vi "task3.vi"() -> ()   [LabVIEW 2021]
panel:
  out "Phase, Freq":cluster{i32[], "detected phases (deg)":dbl[]}(graph)
  out "Amp, Freq":cluster{i32[], dbl[]}(graph)
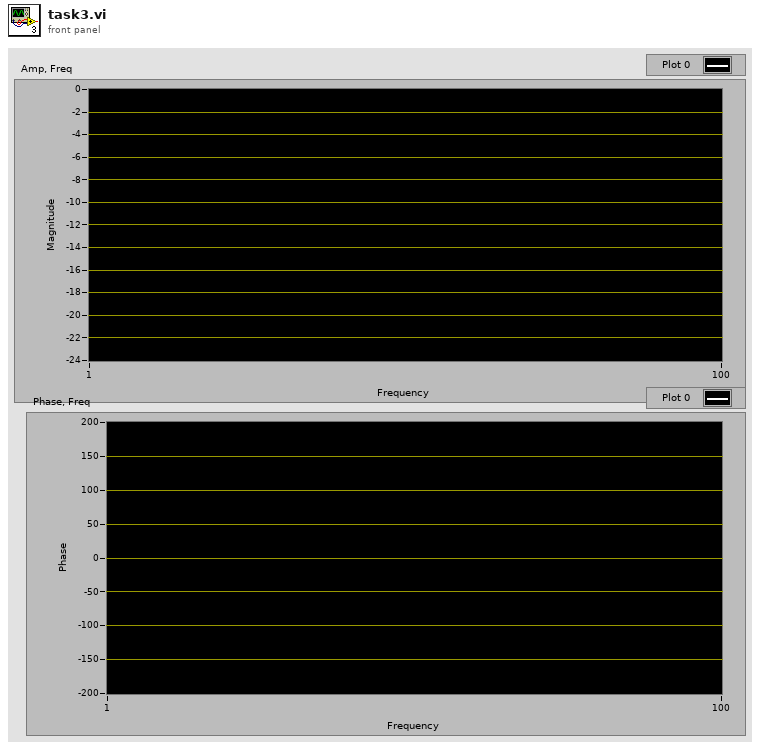
[diagram p1: front panel]
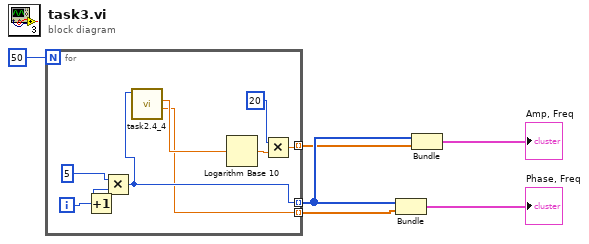
[diagram p0: block diagram]
diagram:
  n1 = for {
    N: 50 -> [_]
    tunnel: [w9] -> w5 mode=indexing
    tunnel: [w10] -> w3 mode=indexing
    tunnel: [w7] -> w2 mode=indexing
    i -> [w15]
    n2 = Increment(x=w15) -> (x+1=w14:i32)
    n3 = Multiply(x=5, y=w14) -> (x*y=w9:i32)
    n4 = call "task2.4_4.vi"("Frequency"=w9) -> ("A1 phase (deg)"=w7:dbl, "A1 amplitude (db)"=w8:dbl)  [unwired: 8 in, 1 out]
    n5 = Logarithm Base 10(1:w8) -> (0:w12:dbl)
    n6 = Multiply(x=20, y=w12) -> (x*y=w10:dbl)
  }
  n7 = Bundle(w5, w2) -> (→"Phase, Freq":cluster{i32[], dbl[]})  [unwired: 1 in]
  n8 = Bundle(w5, w3) -> (→"Amp, Freq":cluster{i32[], dbl[]})  [unwired: 1 in]
